vi "IF_AF.vi"() -> ()   [LabVIEW 2016]
uses:
  <vilib>/Analysis/baseanly.llb/Mean (DBL).vi
  <vilib>/ULx/Create Channel.llb/ULx Create Channel (AI-Voltage-Basic).vi
  <vilib>/ULx/Timing.llb/ULx Timing (Sample Clock).vi
  <vilib>/ULx/Read.llb/ULx Read (Analog 1D Wfm NChan NSamp).vi
  <vilib>/Waveform/WDTOps.llb/WDT Index Channel DBL.vi
  <vilib>/Analysis/NI_AALBase.lvlib
panel:
  out "Flow Rate (SLPS)":dbl
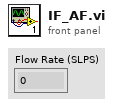
[diagram p1: front panel]
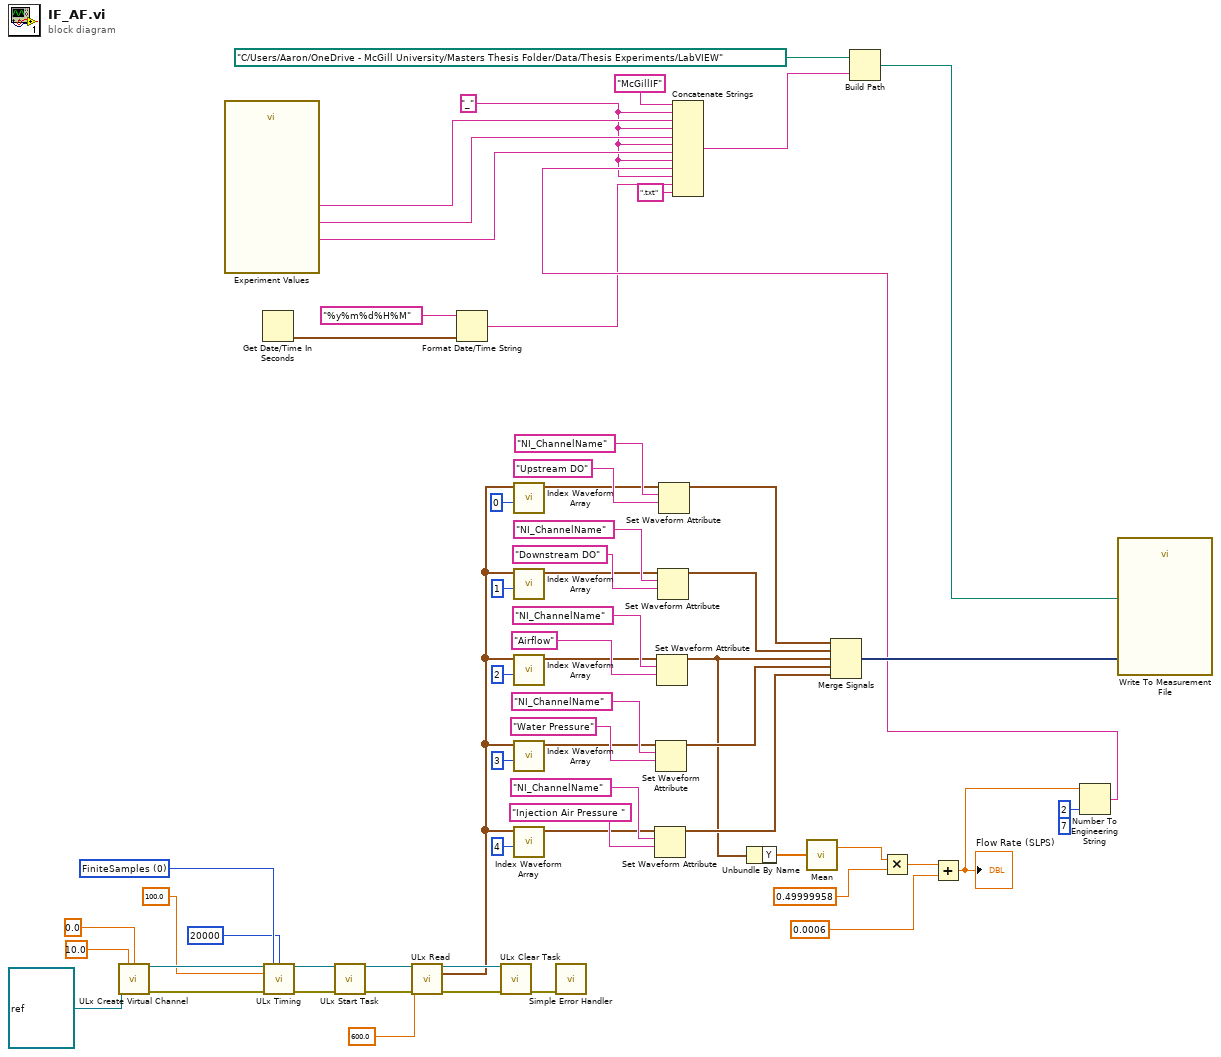
[diagram p0: block diagram]
diagram:
  (unwired) i16 7 ("width (-)")
  w5 = "_"
  w51 = 0 items=["FiniteSamples", "ContinuousSamples"] ("sample mode")
  n1 = call-poly <vilib>:"ULx Create Virtual Channel.vi"("maximum value"=10.0, "minimum value"=0.0, "physical channels"=refnum<k21> "Dev0/Ai0:1, Dev0/Ai7:5") -> ("task out"=w63:refnum<k24>, "error out"=w59:errorcluster)  [unwired: 11 in]
  n2 = call "Experiment Values"() -> ("Water Temperature (C)"=w15:string, "Atmospheric Air Pressure (kPa)"=w16:string, "Water Flowrate (gpm)"=w17:string)  [unwired: 15 in, 2 out]
  n3 = Get Date/Time In Seconds() -> (seconds since 1Jan1904=w20:timestamp)
  n4 = call-poly <vilib>:"ULx Timing.vi"("task in"=w63, "sample mode"=w51, "samples per channel"=20000, "rate"=100.0, "error in"=w59) -> ("task out"=w62:refnum<k24>, "error out"=w58:errorcluster)  [unwired: 9 in]
  n5 = call <vilib>:"ULx Start Task.vi"("task in"=w62, "error in"=w58) -> ("task out"=w61:refnum<k24>, "error out"=w57:errorcluster)  [unwired: 12 in]
  n6 = call-poly <vilib>:"ULx Read.vi"("task in"=w61, "timeout"=600.0, "error in"=w57) -> ("task out"=w60:refnum<k24>, "data"=w44:waveform(dbl)[], "error out"=w56:errorcluster)  [unwired: 10 in]
  n7 = Format Date/Time String(time format string (%c)="%y%m%d%H%M", seconds (now)=w20) -> (date/time string=w4:string)  [unwired: 1 in]
  n8 = call <vilib>:"ULx Clear Task.vi"("task in"=w60, "error in"=w56) -> ("error out"=w55:errorcluster)  [unwired: 13 in]
  n9 = call-poly <vilib>:"Index Waveform Array.vi"("index"=0, "waveform array"=w44) -> ("waveform"=w41:waveform(dbl))  [unwired: 8 in, 1 out]
  n10 = call-poly <vilib>:"Index Waveform Array.vi"("index"=1, "waveform array"=w44) -> ("waveform"=w38:waveform(dbl))  [unwired: 8 in, 1 out]
  n11 = call-poly <vilib>:"Index Waveform Array.vi"("index"=2, "waveform array"=w44) -> ("waveform"=w35:waveform(dbl))  [unwired: 8 in, 1 out]
  n12 = call-poly <vilib>:"Index Waveform Array.vi"("index"=3, "waveform array"=w44) -> ("waveform"=w32:waveform(dbl))  [unwired: 8 in, 1 out]
  n13 = call-poly <vilib>:"Index Waveform Array.vi"("index"=4, "waveform array"=w44) -> ("waveform"=w29:waveform(dbl))  [unwired: 8 in, 1 out]
  n14 = call <vilib>:"Simple Error Handler.vi"("error in (no error)"=w55) -> ()  [unwired: 4 in, 5 out]
  n15 = Set Waveform Attribute(5:"Injection Air Pressure ", 6:"NI_ChannelName" ("name"), 7:w29) -> (3:w25:waveform(dbl))  [unwired: 1 in, 2 out]
  n16 = Set Waveform Attribute(5:"Water Pressure", 6:"NI_ChannelName" ("name"), 7:w32) -> (3:w26:waveform(dbl))  [unwired: 1 in, 2 out]
  n17 = Set Waveform Attribute(5:"Airflow", 6:"NI_ChannelName" ("name"), 7:w35) -> (3:w7:waveform(dbl))  [unwired: 1 in, 2 out]
  n18 = Set Waveform Attribute(5:"Downstream DO", 6:"NI_ChannelName" ("name"), 7:w38) -> (3:w27:waveform(dbl))  [unwired: 1 in, 2 out]
  n19 = Set Waveform Attribute(5:"Upstream DO", 6:"NI_ChannelName" ("name"), 7:w41) -> (3:w28:waveform(dbl))  [unwired: 1 in, 2 out]
  n20 = Unbundle By Name(w7) -> ("Y"=w8:dbl[])
  n21 = call-poly <vilib>:"Mean.vi"("X"=w8) -> ("mean"=w14:dbl)  [unwired: 1 out]
  n22 = Merge Signals(w28, w27, w7, w26, w25) -> (w24:dynamicdata)
  n23 = Multiply(x=w14, y=0.49999958) -> (x*y=w12:dbl)
  n24 = Add(x=w12, y=0.0006) -> (x+y=w9:dbl)
  "Flow Rate (SLPS)" <- w9
  n25 = Number To Engineering String(2:i16 2 ("precision (6)"), 4:w9) -> (0:w6:string)  [unwired: 2 in]
  n26 = Concatenate Strings("McGillIF", w5, w17, w5, w16, w5, w15, w5, w6, w5, w4, ".txt" ("string")) -> (w21:string)
  n27 = Build Path(base path=path "C:/Users/Aaron/OneDrive - McGill University/Masters Thesis Folder/Data/Thesis Experiments/LabVIEW" ("Filename"), name or relative path=w21) -> (appended path=w22:path)
  n28 = call "Write To Measurement File"("Signals"=w24, "Filename"=w22) -> ()  [unwired: 15 in, 3 out]
